vi "poly_wait_for_value_change_multi.vi"(6 "timeout (never)":i32=-1, 8 "error in":errorcluster, 9 "stop ref":refnum<vi>, 10 "control ref":refnum<vi>[](array[refnum])) -> (0 "error out":errorcluster, 2 "timed out?":bool)   [LabVIEW 2015]
panel:
  out "stop?":bool
  in  "dummy stop":bool
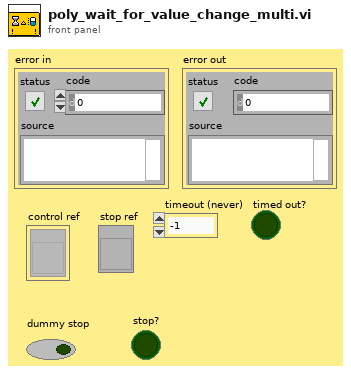
[diagram p1: front panel]
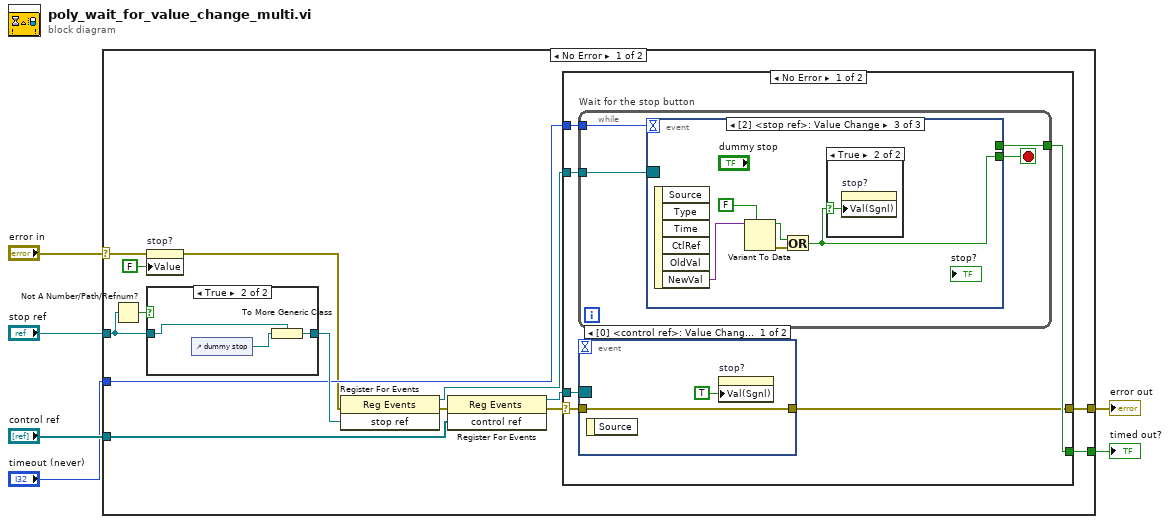
[diagram p0: block diagram]
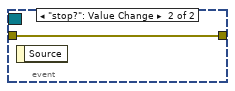
[diagram p2: hidden frame]
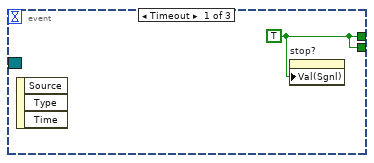
[diagram p3: hidden frame]
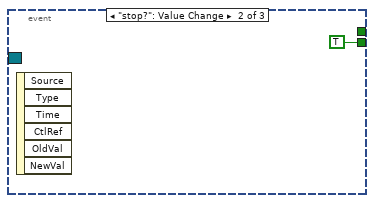
[diagram p4: hidden frame]
diagram:
  n1 = case shown="No Error" "error in" {
    selector: "error in" -> [w13 w47]
    tunnel: "control ref" -> [w18 _]
    tunnel: [w8 w47] -> w4
    tunnel: "stop ref" -> [w19 _]
    tunnel: "timeout (never)" -> [w15 _]
    tunnel: [w11 _] -> w1
    frame No Error {
      n2 = Not A Number/Path/Refnum?(number/path/refnum=w19) -> (NaN/Path/Refnum?=w20:bool)
      n3 = property on="stop?" class="Bool (strict)"(error in=w13, "Value"=FALSE ("stop?")) -> (error out=w12:errorcluster)  [unwired: 1 in, 1 out]
      n4 = case shown="True" w20 {
        tunnel: w19 -> [w43 w45]
        tunnel: [w43 w44] -> w17
        frame False {
        }
        frame True {
          n5 = control-ref of="dummy stop"() -> (w46:refnum<vi>)
          n6 = To More Generic Class(target class=w45, reference=w46) -> (generic class reference=w44:refnum<vi>)
        }
      }
      n7 = register-events(error in=w12, w17) -> (reference out=w16:refnum<event-registration>, error out=w10:errorcluster)  [unwired: 1 in]
      n8 = register-events(error in=w10, w18) -> (reference out=w7:refnum<event-registration>, error out=w9:errorcluster)  [unwired: 1 in]
      n9 = case shown="No Error" w9 {
        selector: w9 -> [w23 w42]
        tunnel: w16 -> [w26 _]
        tunnel: w15 -> [w25 _]
        tunnel: [w24 _] -> w11
        tunnel: [w22 w42] -> w8
        tunnel: w7 -> [w21 _]
        frame No Error {
          n10 = while "Wait for the stop button" {
            tunnel: w26 -> [w33]
            tunnel: w25 -> [w30]
            tunnel: [w31] -> w24
            stop <- w32 stop-if-true
            n11 = event shown="[2] <stop ref>: Value Change" {
              selector: w33 -> [_ _ _]
              dyn-events: _ -> [_ _ _]
              timeout: w30 -> [_ _ _]
              tunnel: [w34 TRUE w36] -> w32
              tunnel: [w34 _ _] -> w31
              event Timeout {
                w34 = TRUE
                n12 = event-data() -> ()  [unwired: 1 in, 3 out]
                n13 = property on="stop?" class="Bool (strict)"("Val(Sgnl)"=w34) -> ()  [unwired: 2 in, 2 out]
              }
              event "stop?": Value Change {
                n14 = event-data() -> ()  [unwired: 1 in, 6 out]
              }
              event Value Change {
                n15 = event-data() -> ("NewVal"=w37:variant)  [unwired: 1 in, 5 out]
                n16 = Variant To Data(type=FALSE, Variant=w37) -> (data=w39:bool, error out=w40:errorcluster)  [unwired: 1 in]
                n17 = Or(x=w39, y=w40) -> (x .or. y?=w36:bool)
                n18 = case shown="True" w36 {
                  selector: w36 -> [_ w41]
                  frame False {
                  }
                  frame True {
                    n19 = property on="stop?" class="Bool (strict)"("Val(Sgnl)"=w41) -> ()  [unwired: 2 in, 2 out]
                  }
                }
              }
            }
          }
          n20 = event shown="[0] <control ref>: Value Change" {
            selector: w21 -> [_ _]
            dyn-events: _ -> [_ _]
            timeout: _ -> [_ _]
            tunnel: [w28 w29] -> w22
            tunnel: w23 -> [w28 w29]
            event Value Change {
              n21 = event-data() -> ()  [unwired: 1 in, 1 out]
              n22 = property on="stop?" class="Bool (strict)"("Val(Sgnl)"=TRUE) -> ()  [unwired: 2 in, 2 out]
            }
            event "stop?": Value Change {
              n23 = event-data() -> ()  [unwired: 1 in, 1 out]
            }
          }
        }
        frame Error {
        }
      }
    }
    frame Error {
    }
  }
  "error out" <- w4
  "timed out?" <- w1
